vi "Count TX-RX samples.vi"(8 "reset":bool, 10 "RX samples":u64, 11 "TX samples":u64) -> (0 "terminal count":bool, 3 "is TX":bool)   [LabVIEW 2020]
uses:
  <instrlib>/_niInstr/Basic Elements/v1/FPGA/Private/Count Down U64.vi
  <instrlib>/_niInstr/Basic Elements/v1/FPGA/niInstr Basic Elements v1 FPGA.lvlib
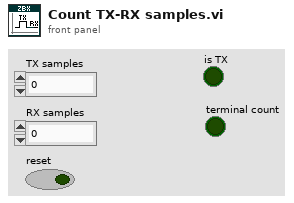
[diagram p1: front panel]
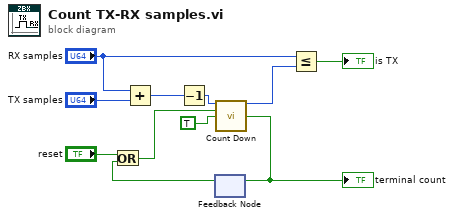
[diagram p0: block diagram]
diagram:
  n1 = Add(x="RX samples", y="TX samples") -> (x+y=w1:u64)
  n2 = Decrement(x=w1) -> (x-1=w2:u64)
  n3 = feedback #1() -> (w4:bool)  [unwired: 1 in]
  n4 = Or(x="reset", y=w4) -> (x .or. y?=w5:bool)
  n5 = call-poly <instrlib>:"Count Down.vi"("count in"=w2, "load"=w5, "decrement"=TRUE) -> ("count out"=w7:u64, "terminal count"=w9:bool)  [unwired: 11 in]
  "terminal count" <- w9
  n6 = feedback-in #1(w9) -> ()
  n7 = Less Or Equal?(x="RX samples", y=w7) -> (x <= y?=→"is TX":bool)
